vi "Project - Memory.vi"(5 "Memory":T1, 7 "Msg Chain":string, 8 "error in (no error)":errorcluster {"code" format="Error %.0f"}, 10 "Project Doc":refnum<class "Project Documentation.lvclass">, 11 "VIDoc Printer In":refnum<class "VIDoc Printer.lvclass">) -> (0 "error out":errorcluster {"code" format="Error %.0f"}, 3 "VIDoc Printer Out":refnum<class "VIDoc Printer.lvclass">)   [LabVIEW 2023, in "VIDoc Printer.lvlib" / "VIDoc Printer.lvclass"]
uses:
  VIDoc Printer.lvclass
  Parsing/Project Documentation/Project Documentation.lvclass
  Parsing/TypeDefs/Memory Size Cluster.ctl
  VIDoc Printer.lvclass/VIDoc Printer.ctl
  Parsing/VIDoc Parsing.lvlib
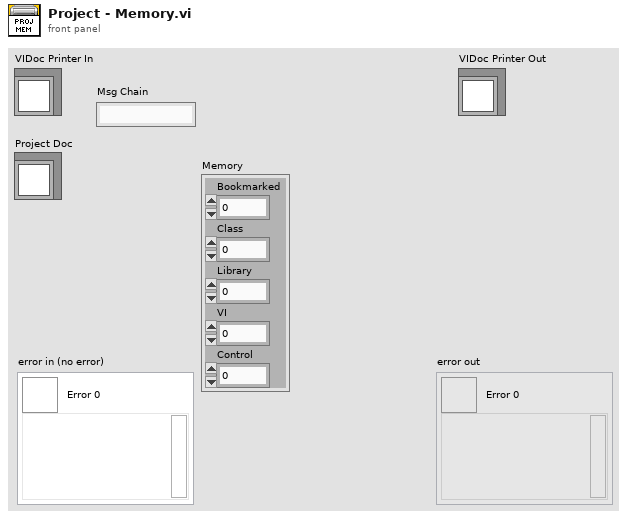
[diagram p1: front panel]
types:
  T1 = typedef "VIDoc Parsing.lvlib/Memory Size Cluster.ctl" = cluster{"Bookmarked":dbl, "Class":dbl, "Library":dbl, "VI":dbl, "Control":dbl}
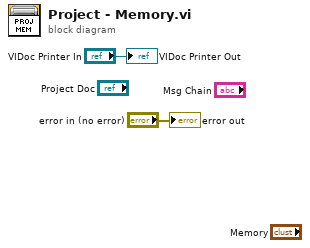
[diagram p0: block diagram]
diagram:
  "error out" <- "error in (no error)"
  "VIDoc Printer Out" <- "VIDoc Printer In"
